vi "Turn Power On Command.vi"(8 "error in (no error)":errorcluster, 10 "EUI Events.lvclass":refnum<class "EUI Events.lvclass">, 11 "command_TurnPowerOn":T1) -> (0 "error out":errorcluster)   [LabVIEW 2016, in "M1M3SupportEUI_Views.lvlib"]
uses:
  M1M3SupportEUI_Views.lvlib
  SALLV_m1m3/DataTypes/command_TurnPowerOn.ctl
  EUI Events/EUI Events.lvclass
  SALLV_m1m3/SALLV_m1m3.lvlib
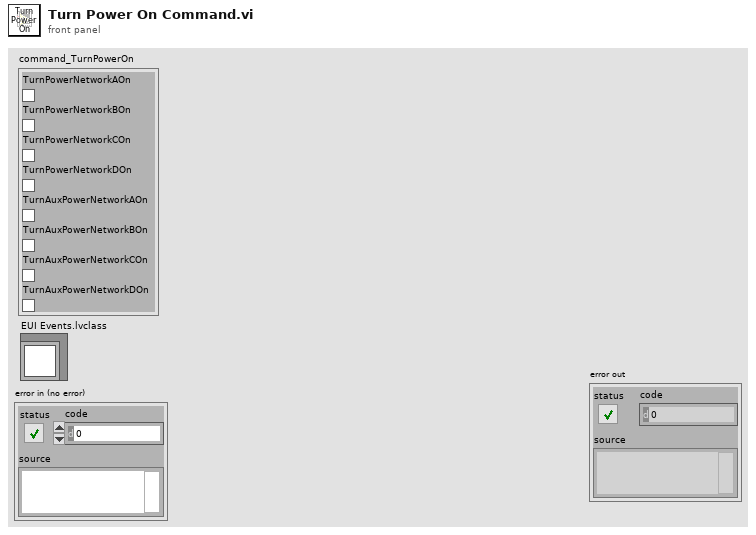
[diagram p1: front panel]
types:
  T1 = typedef "SALLV_m1m3.lvlib/command_TurnPowerOn.ctl" = cluster{"TurnPowerNetworkAOn":bool, "TurnPowerNetworkBOn":bool, "TurnPowerNetworkCOn":bool, "TurnPowerNetworkDOn":bool, "TurnAuxPowerNetworkAOn":bool, "TurnAuxPowerNetworkBOn":bool, "TurnAuxPowerNetworkCOn":bool, "TurnAuxPowerNetworkDOn":bool}
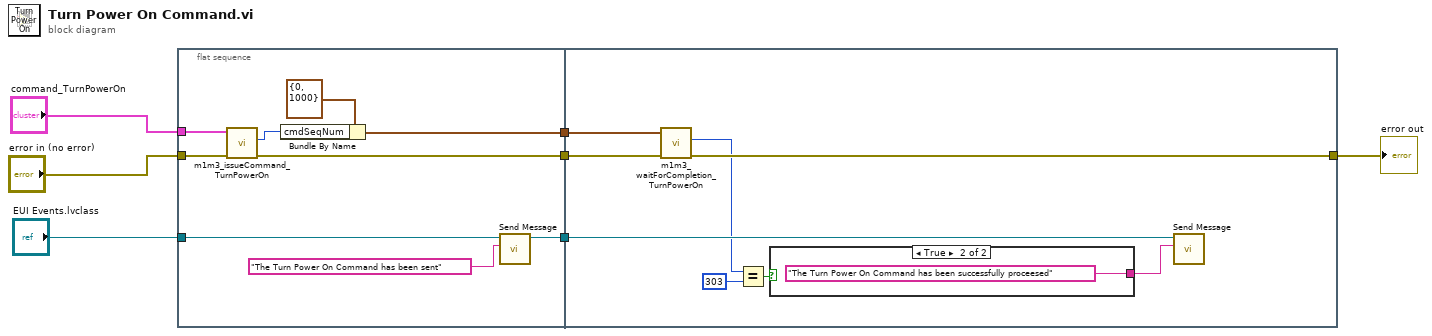
[diagram p0: block diagram]
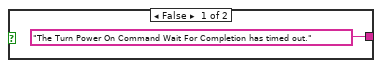
[diagram p2: hidden frame]
diagram:
  n1 = flat-sequence {
    tunnel: "command_TurnPowerOn" -> [w14]
    tunnel: "error in (no error)" -> [w13]
    tunnel: "EUI Events.lvclass" -> [w11]
    tunnel: [w9] -> w3
    tunnel: [w10] -> w2
    tunnel: [w8] -> w1
    tunnel: [w23] -> w5
    tunnel: w3 -> [w23]
    tunnel: w2 -> [w19]
    tunnel: w1 -> [w18]
    frame #0 {
      n2 = call "m1m3_issueCommand_TurnPowerOn.vi"("error in (no error)"=w13, "command_TurnPowerOn_Ctl"=w14) -> ("error out"=w9:errorcluster, "function return"=w16:i32)  [unwired: 7 in, 1 out]
      n3 = Bundle By Name(cluster=cluster{"cmdSeqNum":i32, "timeout":u32} {"cmdSeqNum"=0, "timeout"=1000} ("waitComplete_Ctl"), "cmdSeqNum"=w16) -> (w8:cluster{"cmdSeqNum":i32, "timeout":u32})
      n4 = call "Send Message.vi"("Message"="The Turn Power On Command has been sent", "EUI Events in"=w11) -> ("EUI Events out"=w10:refnum<class "EUI Events.lvclass">)  [unwired: 8 in, 1 out]
    }
    frame #1 {
      n5 = call "m1m3_waitForCompletion_TurnPowerOn.vi"("waitComplete_Ctl"=w18) -> ("function return"=w17:i32)  [unwired: 8 in, 2 out]
      n6 = Equal?(x=w17, y=303) -> (x = y?=w21:bool)
      n7 = case shown="True" w21 {
        tunnel: ["The Turn Power On Command Wait For Completion has timed out." ("Message") "The Turn Power On Command has been successfully proceesed" ("Message")] -> w20
        frame False {
        }
        frame True {
        }
      }
      n8 = call "Send Message.vi"("Message"=w20, "EUI Events in"=w19) -> ()  [unwired: 8 in, 2 out]
    }
  }
  "error out" <- w5
